vi "Core Action.vi"(8 "error in (no error)":errorcluster, 10 "SECS-II Class":refnum<class "SECS-II Class.lvclass">, 11 "Establish Communications in":refnum<class "01-Establish Communications.lvclass">) -> (0 "error out":errorcluster, 2 "SECS-II Class Out":refnum<class "SECS-II Class.lvclass">, 3 "Establish Communications out":refnum<class "01-Establish Communications.lvclass">)   [LabVIEW 2020, in "SECS Scenarios.lvlib" / "01-Establish Communications.lvclass"]
uses:
  01-Establish Communications.lvclass
  D:/Dropbox/SECS/SECS_GEM v1.1.0/Com/SECS Scenarios/Scenarios Class/Scenarios Class.lvclass
  SECS Communication/SECS-II Class/SECS-II Class.lvclass
  SECS Communication/S1 Message Class/S1 Message Class.lvclass
  D:/Dropbox/SECS/SECS_GEM v1.1.0/Com/SECS Communication/SECS-II Class/SECS-II Class.lvclass
  Scenarios Class/Reply State.ctl
  Scenarios Class/Scenarios Class.lvclass/Scenarios Class.ctl
  SECS Communication/S1 Message Class/S1F14.ctl
  Scenarios Class/Write Reply State.vi
  Scenarios Class/Read HSMS Class.vi
  SECS Communication/SECS Data Class/Get ECID Data.vi
  SECS Communication/SECS-II Class/Variant To Data_ASCII.vi
  SECS Communication/HSMS Class/HSMS Class.lvclass
  SECS Communication/SECS Data Class/SECS Data Class.lvclass
  Scenarios Class/Scenarios Class.lvclass
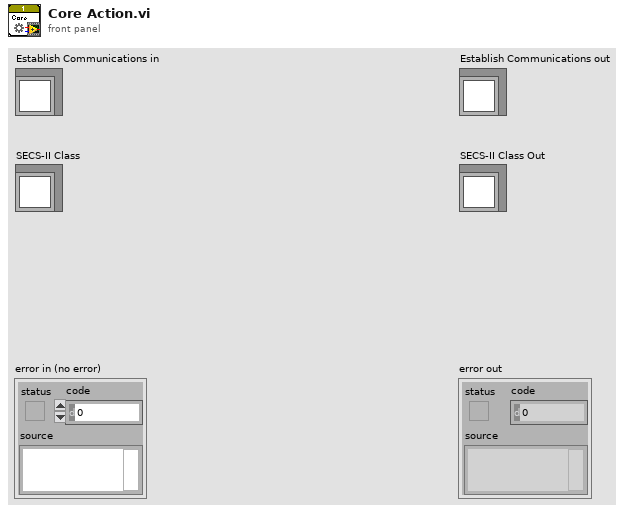
[diagram p1: front panel]
types:
  T1 = typedef "SECS Scenarios.lvlib/Scenarios Class.lvclass/Reply State.ctl" = enum16{"OK", "Illegal Data", "Unknown Stream", "Unknown Function", "Off-Line", "T3 Timeout", "Inner-Timeout"}
  T2 = typedef "SECS Communication.lvlib/S1 Message Class.lvclass/S1F14.ctl" = cluster{"MDLN":string, "SOFTREV":string, "COMMACK":bool}
  T3 = typedef "SECS Communication.lvlib/SECS Data Class.lvclass/ECID Data.ctl" = cluster{"ECID":u32, "Name":string, "Description":string, "Format Code":T4, "Unit":string, "Max":dbl, "Min":dbl, "Default":string, "Source":string, "Data":variant}
  T4 = typedef "SECS Communication.lvlib/SECS-II Class.lvclass/Format Code.ctl" = enum16{"L", "A", "B", "Boolean", "J", "I1", "I2", "I4", "I8", "U1", "U2", "U4", "U8", "F4", "F8", "Char"}
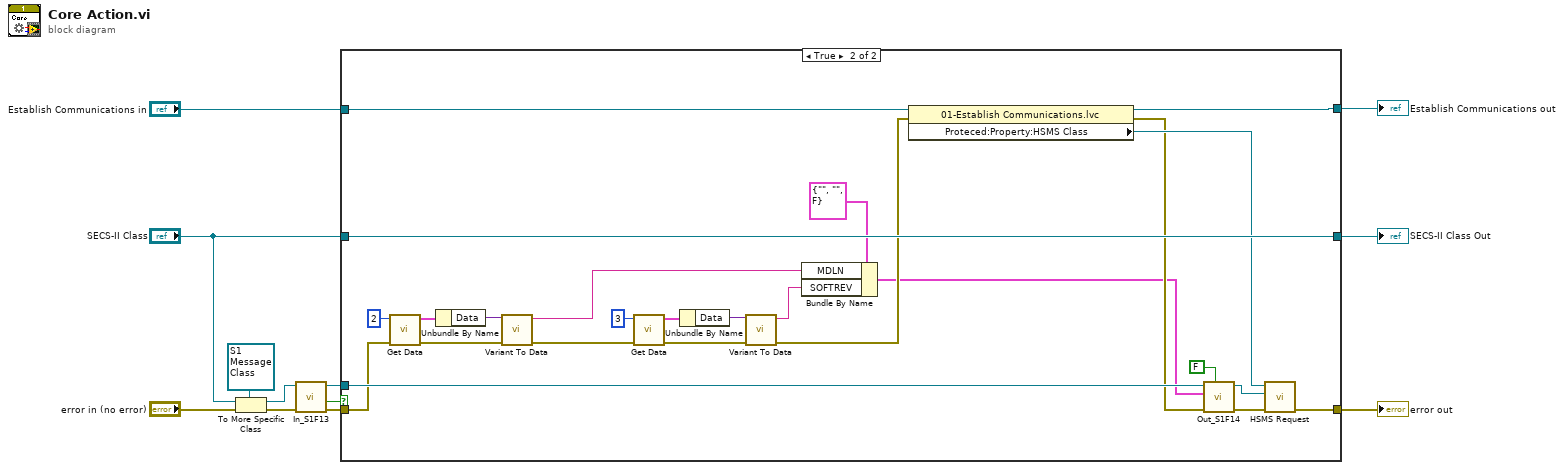
[diagram p0: block diagram]
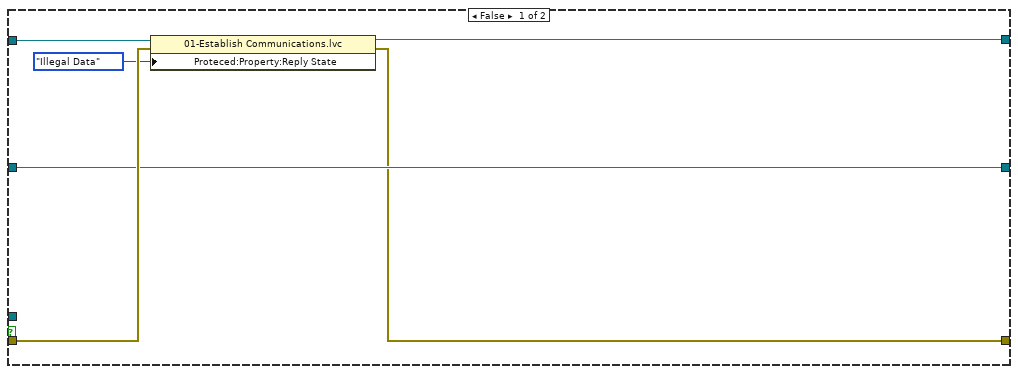
[diagram p2: hidden frame]
diagram:
  n1 = To More Specific Class(target class=refnum<class "S1 Message Class.lvclass"> refnum ("S1 Message Class in"), reference="SECS-II Class", error in="error in (no error)") -> (specific class reference=w10:refnum<class "S1 Message Class.lvclass">, error out=w11:errorcluster)
  n2 = call "In_S1F13.vi"("error in (no error)"=w11, "S1 Message Class in"=w10) -> ("error out"=w8:errorcluster, "OK?"=w6:bool, "S1 Message Class out"=w7:refnum<class "S1 Message Class.lvclass">)  [unwired: 6 in, 1 out]
  n3 = case shown="True" w6 {
    tunnel: [w14 w43] -> w12
    tunnel: w8 -> [w17 w21]
    tunnel: w7 -> [_ w39]
    tunnel: "Establish Communications in" -> [w18 w37]
    tunnel: [w15 w36] -> w5
    tunnel: "SECS-II Class" -> [w16 w38]
    tunnel: [w16 w38] -> w3
    frame False {
      n4 = property class="01-Establish Communications.lvc"(reference=w18, error in=w17, "Proteced:Property:Reply State"=Reply_State."Illegal Data" ("Reply State")) -> (reference out=w15:refnum<class "01-Establish Communications.lvclass">, error out=w14:errorcluster)
    }
    frame True {
      n5 = call-poly "Get Data.vi"("error in"=w21, "ECID"=u32 2) -> ("error out"=w26:errorcluster, "ECID Data"=w25:T3)  [unwired: 7 in, 1 out]
      n6 = Unbundle By Name(w25) -> ("Data"=w27:variant)
      n7 = call-poly "Variant To Data.vi"("error in (no error)"=w26, "Variant"=w27) -> ("error out"=w31:errorcluster, "Data"=w32:string)  [unwired: 7 in, 1 out]
      n8 = call-poly "Get Data.vi"("error in"=w31, "ECID"=u32 3) -> ("error out"=w29:errorcluster, "ECID Data"=w30:T3)  [unwired: 7 in, 1 out]
      n9 = Unbundle By Name(w30) -> ("Data"=w28:variant)
      n10 = call-poly "Variant To Data.vi"("error in (no error)"=w29, "Variant"=w28) -> ("error out"=w20:errorcluster, "Data"=w33:string)  [unwired: 7 in, 1 out]
      n11 = Bundle By Name(cluster=T2 {"MDLN"="", "SOFTREV"="", "COMMACK"=FALSE} ("S1F13"), "MDLN"=w32, "SOFTREV"=w33) -> (w19:T2)
      n12 = property class="01-Establish Communications.lvc"(reference=w37, error in=w20) -> (reference out=w36:refnum<class "01-Establish Communications.lvclass">, error out=w34:errorcluster, "Proteced:Property:HSMS Class"=w35:refnum<class "HSMS Class.lvclass">)
      n13 = call "Out_S1F14.vi"("Host"=FALSE, "error in (no error)"=w34, "S1F14"=w19, "S1 Message Class in"=w39) -> ("error out"=w41:errorcluster, "S1 Message Class out"=w40:refnum<class "S1 Message Class.lvclass">)  [unwired: 6 in]
      n14 = call "HSMS Request.vi"("error in (no error)"=w41, "SECS-II Class In"=w40, "HSMS Class in"=w35) -> ("error out"=w43:errorcluster)  [unwired: 7 in, 1 out]
    }
  }
  "error out" <- w12
  "Establish Communications out" <- w5
  "SECS-II Class Out" <- w3
